vi "SVN_NumberToRevCommand.vi"(11 "rev End":i32) -> (3 "String":string)   [LabVIEW 2014]
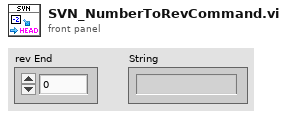
[diagram p1: front panel]
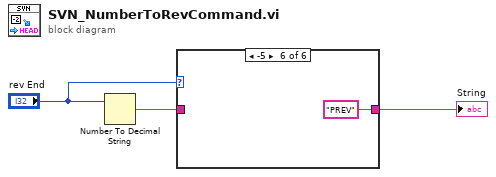
[diagram p0: block diagram]
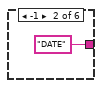
[diagram p3: hidden frame]
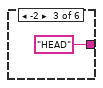
[diagram p4: hidden frame]
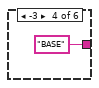
[diagram p5: hidden frame]
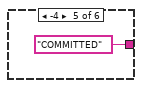
[diagram p6: hidden frame]
diagram:
  n1 = Number To Decimal String(number="rev End") -> (decimal integer string=w1:string)  [unwired: 1 in]
  n2 = case shown="-5" "rev End" {
    tunnel: w1 -> [w4 _ _ _ _ _]
    tunnel: [w4 "DATE" "HEAD" "BASE" "COMMITTED" "PREV"] -> w3
    frame 0.., Default {
    }
    frame -1 {
    }
    frame -2 {
    }
    frame -3 {
    }
    frame -4 {
    }
    frame -5 {
    }
  }
  "String" <- w3
